vi "ADAM_Hi-Tec_convert.vi"(0 "Ch Name":string, 1 "Raw":dbl format="%.3f") -> (5 "Q release (l/min)":dbl format="%.2f", 6 "M_dot (kg/min)":dbl format="%.4f", 7 "Comments":string)   [LabVIEW 2010]
uses:
  Anemometry/Anemometry Sub Vis/Globals/Gas_management_global.vi
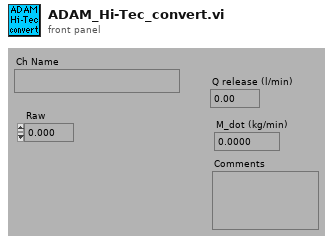
[diagram p1: front panel]
types:
  T1 = enum16{"Q(release) to Volts", "Volts to Q(release)"}
  T2 = typedef "Hi-Tec_calib.ctl" = cluster{"Ref temp (deg C)":dbl, "Ref Pres (mbars)":dbl, "Density at calib conditions":dbl, "Coefficients":dbl[]}
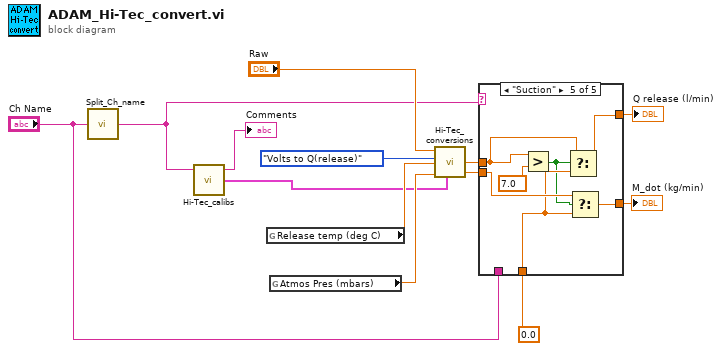
[diagram p0: block diagram]
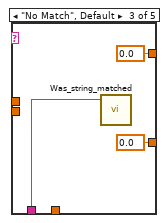
[diagram p4: hidden frame]
diagram:
  n1 = call "Split_Ch_name.vi"("Ch name"="Ch Name") -> ("Middle"=w3:string)  [unwired: 2 out]
  n2 = call "Hi-Tec_calibs.vi"("Gas Line Name"=w3) -> ("Hi-Tec calib"=w5:T2, "Comments"=→"Comments":string)  [unwired: 3 out]
  n3 = global read "Gas_management_global.vi" "Release temp (deg C)"() -> (w12:dbl)
  n4 = global read "Gas_management_global.vi" "Atmos Pres (mbars)"() -> (w11:dbl)
  n5 = call "Hi-Tec_conversions.vi"("Input"="Raw", "Conversion"=T1."Volts to Q(release)", "Release temp (deg C)"=w12, "Atmos Pres (mbars)"=w11, "Hi-Tec calib"=w5) -> ("Output"=w9:dbl, "Flowrate (kg/min)"=w7:dbl)  [unwired: 1 out]
  n6 = case shown="\"Suction\"" w3 {
    tunnel: w9 -> [w15 w17 _ w22 w25]
    tunnel: [w15 w17 0.0 ("Output") w22 w29] -> w8
    tunnel: w7 -> [w14 w16 _ w21 w28]
    tunnel: [w14 w16 0.0 ("Flowrate (kg/min)") w21 w27] -> w6
    tunnel: 0.0 -> [_ _ _ _ w26]
    tunnel: "Ch Name" -> [_ _ w20 _ _]
    frame "Carrier 1" {
    }
    frame "Carrier 2" {
    }
    frame "No Match", Default {
      n7 = call "Was_string_matched.vi"("Variable name"=w20) -> ()  [unwired: 2 in]
    }
    frame "Trace" {
    }
    frame "Suction" {
      n8 = Greater?(x=w25, y=7.0) -> (0:w24:bool)
      n9 = Select(t=w25, s=w24, f=w26) -> (s? t:f=w29:dbl)
      n10 = Select(t=w28, s=w24, f=w26) -> (s? t:f=w27:dbl)
    }
  }
  "Q release (l/min)" <- w8
  "M_dot (kg/min)" <- w6
